vi "Compiled Get Node Settings.vi"(8 "error in":errorcluster, 10 "Cluster":refnum<k21>, 11 "Addon Ref":T21 format="%.0x") -> (0 "error out":errorcluster, 2 "J1939 Data Settings":T1 {"Monitor"."Data"."Outgoing"."Trigger.Refs"."Data Reference" format="%.0x"; "Monitor"."Data"."Outgoing"."Disable.Refs"."Data Reference" format="%.0x"; "Monitor"."Data"."Outgoing"."Data.Refs"."Data Reference" format="%.0x"; "Monitor"."Data"."Incoming"."Timing.Refs"."Data Reference" format="%.0x"; "Monitor"."Data"."Incoming"."Data.Refs"."Data Reference" format="%.0x"; "Monitor"."Network"."Name" format="%.0x"; "Sim"."DTCs"."DM1.Ref"."Data Reference" format="%.0x"; "Sim"."DTCs"."DM1.Enable.Ref"."Data Reference" format="%.0x"; "Sim"."DTCs"."DM2.Ref"."Data Reference" format="%.0x"; "Sim"."DTCs"."DM2.Enable.Ref"."Data Reference" format="%.0x"; "Sim"."Network"."Name" format="%.0x"}, 3 "Addon Ref out":T21=18446744073709551615 format="%.0x")   [LabVIEW 2023, in "J1939 Addon System Explorer.lvlib"]
uses:
  J1939 Addon System Explorer.lvlib
  <vilib>/NI VeriStand/Custom Device API/Custom Device Item Ref.ctl
  Addon Shared/Types/Compiled.Node Settings.ctl
  Addon Shared/Types/Compiled Monitor Tool Settings.ctl
  Addon Shared/Types/Monitor Settings.ctl
  Addon Shared/Types/Device Settings.ctl
  Addon Shared/Types/Incoming Settings.ctl
  Addon Shared/Types/Incoming Frame Settings.ctl
  <vilib>/NI VeriStand/Custom Device API/Block Data Reference.ctl
  <vilib>/NI VeriStand/Custom Device API/Data Reference.ctl
  Addon Shared/Types/Outgoing Settings.ctl
  Addon Shared/Types/Outgoing Frame Settings.ctl
  Addon Shared/Types/Outgoing Event Trigger Types.ctl
  SubModules/Frame-Protection-Support/Source/Shared/Types/Exported Frame Settings.ctl
  SubModules/Frame-Protection-Support/Source/Shared/Types/Exported Frame Type.ctl
  SubModules/Frame-Protection-Support/Source/Shared/Types/Exported Protection Settings.ctl
  SubModules/Frame-Protection-Support/Source/Shared/Types/Protection Type.ctl
  SubModules/Frame-Protection-Support/Source/Shared/Types/XNET Signal Configuration.ctl
  SubModules/Frame-Protection-Support/Source/Shared/Types/Exported Counter Settings.ctl
  SubModules/Frame-Protection-Support/Source/Shared/Types/Exported Event Trigger Type.ctl
  Addon Shared/Types/Complied Simulated Device Settings.ctl
  Addon Shared/Types/Compiled Simulated Settings.ctl
  Addon Shared/J1939 Addon Shared.lvlib
  <vilib>/NI VeriStand/Custom Device API/Custom Device API.lvlib
  <vilib>/NI/NIVS Inline Async API/_Data Access System Explorer/Data Access System Explorer.lvlib
  SubModules/Frame-Protection-Support/Source/Shared/Protection and Counter Support Shared.lvlib
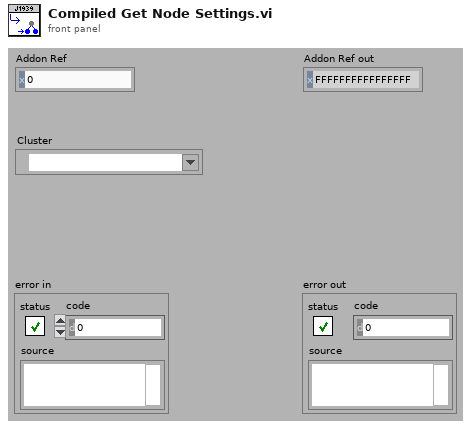
[diagram p1: front panel]
types:
  T1 = typedef "J1939 Addon Shared.lvlib/Compiled.Node Settings.ctl" = cluster{"Monitor":T2, "Sim":T19[]}
  T2 = typedef "J1939 Addon Shared.lvlib/Compiled Monitor Tool Settings.ctl" = cluster{"Network":T3, "Data":T4}
  T3 = typedef "J1939 Addon Shared.lvlib/Monitor Settings.ctl" = cluster{"Address":u8, "Name":u64, "Include DA":bool, "Force SA":bool}
  T4 = typedef "J1939 Addon Shared.lvlib/Device Settings.ctl" = cluster{"Incoming":T5, "Outgoing":T9}
  T5 = typedef "J1939 Addon Shared.lvlib/Incoming Settings.ctl" = cluster{"Signals":string[], "Frames":T6[], "Data.Refs":T7[], "Data.Values":dbl[], "Timing.Use":bool, "Timing.Refs":T7[], "Timing.Values":dbl[], "Timing.Index":i32[]}
  T6 = typedef "J1939 Addon Shared.lvlib/Incoming Frame Settings.ctl" = cluster{"Signals":string[], "PGN":u32}
  T7 = typedef "Custom Device API.lvlib/Block Data Reference.ctl" = cluster{"Data Reference":T8, "Offset":u64, "Length":u64}
  T8 = typedef "Custom Device API.lvlib/Data Reference.ctl" = i32
  T9 = typedef "J1939 Addon Shared.lvlib/Outgoing Settings.ctl" = cluster{"Frames":T10[], "Data.Refs":T7[], "Data.Values":dbl[], "Disable.Refs":T7[], "Disable.Values":dbl[], "Trigger.Refs":T7[], "Trigger.Values":dbl[], "Frames.CountersAndProtections":T12[]}
  T10 = typedef "J1939 Addon Shared.lvlib/Outgoing Frame Settings.ctl" = cluster{"Signals":string[], "Channel Array Position":cluster{"Offset":u32, "Length":u32}, "PGN":u32, "Cyclic?":bool, "Disable?":bool, "Disable.Index":i32, "Trigger":T11, "Trigger.Index":i32}
  T11 = typedef "J1939 Addon Shared.lvlib/Outgoing Event Trigger Types.ctl" = enum16{"Channel value change", "Trigger channel (not zero)", "Channel value change or trigger channel (not zero)", "Trigger channel (any value change)", "Channel value change or trigger channel (any value change)"}
  T12 = typedef "Protection and Counter Support Shared.lvlib/Exported Frame Settings.ctl" = cluster{"Type":T13, "Frame ID":u32, "Payload Length":u32, "Signal XNET Paths":string[], "Frame.PrevData":dbl[], "VS Offset":i32, "VS Length":i32, "Generation Period":u32, "Has Protection?":bool, "Protection Configurations":T14[], "Has Counter":bool, "Counter Configurations":T17[], "Has Disable?":bool, "Disable VS Index":i32, "Transmit Trigger":T18, "Trigger VS Index":i32}
  T13 = typedef "Protection and Counter Support Shared.lvlib/Exported Frame Type.ctl" = enum16{"Periodic", "Event", "Periodic/Event"}
  T14 = typedef "Protection and Counter Support Shared.lvlib/Exported Protection Settings.ctl" = cluster{"Protection Frame Index":i32, "Protection Type":T15, "Data Indeces":i32[], "Initialized Data Array":dbl[], "Protection Signal XNET Paths":string[], "CRC Channels":T16[], "Protection VS Update Index":i32, "Override Index":i32, "Override Value Index":i32}
  T15 = typedef "Protection and Counter Support Shared.lvlib/Protection Type.ctl" = enum16{"Arb ID + Bytes Checksum with Inversion", "Arb ID + Bytes CRC with Inversion", "Reversed Raw Signal Checksum with Inversion", "Concatenated Two's Compliment"}
  T16 = typedef "Protection and Counter Support Shared.lvlib/XNET Signal Configuration.ctl" = cluster{"Start Bit":i32, "Name":string, "Number of bits":i32, "Scale":dbl, "Offset":dbl, "Data Type":u32, "Counter":bool}
  T17 = typedef "Protection and Counter Support Shared.lvlib/Exported Counter Settings.ctl" = cluster{"Frame Index":i32, "Max Count":dbl, "VS Index":i32, "Bit Length":i64, "Override Index":i32, "Override Value Index":i32}
  T18 = typedef "Protection and Counter Support Shared.lvlib/Exported Event Trigger Type.ctl" = enum16{"Channel value change", "Trigger channel (not zero)", "Channel value change or trigger channel (not zero)", "Trigger channel (any value change)", "Channel value change or trigger channel (any value change)"}
  T19 = typedef "J1939 Addon Shared.lvlib/Complied Simulated Device Settings.ctl" = cluster{"Network":T3, "Data":T4, "DTCs":T20}
  T20 = typedef "J1939 Addon Shared.lvlib/Compiled Simulated Settings.ctl" = cluster{"DM1.Ref":T7[], "DM1.Value":dbl[], "DM1.Enable.Ref":T7[], "DM1.Enable.Value":dbl[], "DM2.Ref":T7[], "DM2.Value":dbl[], "DM2.Enable.Ref":T7[], "DM2.Enable.Value":dbl[]}
  T21 = typedef "Custom Device API.lvlib/Custom Device Item Ref.ctl" = u64
  T22 = cluster{"Name":string, "Type":enum16{"Output/Write", "Input/Read", "Input/ReadWrite"}, "VS Refs":T21[]}[]
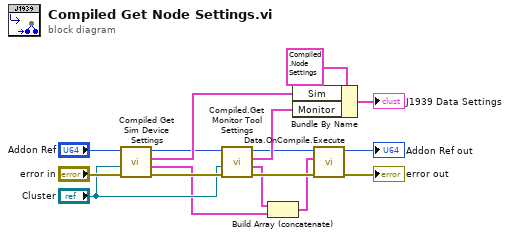
[diagram p0: block diagram]
diagram:
  n1 = call "Compiled Get Sim Device Settings.vi"("error in (no error)"="error in", "Cluster"="Cluster", "Addon Ref"="Addon Ref") -> ("error out"=w11:errorcluster, "Async Refs"=w3:T22, "Settings"=w13:T19[], "Addon Ref out"=w8:T21)  [unwired: 5 in]
  n2 = call "Compiled.Get Monitor Tool Settings.vi"("error in (no error)"=w11, "Cluster"="Cluster", "Addon Ref"=w8) -> ("error out"=w7:errorcluster, "VS Ref Groups"=w2:T22, "MonitorToolSettings"=w10:T2, "Addon Ref out"=w5:T21)  [unwired: 5 in]
  n3 = Build Array (concatenate)(w2, w3) -> (w1:T22)
  n4 = Bundle By Name(cluster=T1 {"Monitor"={"Network"={"Address"=0, "Name"=0, "Include DA"=FALSE, "Force SA"=FALSE}, "Data"={"Incoming"={"Signals"=[], "Frames"=[], "Data.Refs"=[], "Data.Values"=[], "Timing.Use"=FALSE, "Timing.Refs"=[], "Timing.Values"=[], "Timing.Index"=[]}, "Outgoing"={"Frames"=[], "Data.Refs"=[], "Data.Values"=[], "Disable.Refs"=[], "Disable.Values"=[], "Trigger.Refs"=[], "Trigger.Values"=[], "Frames.CountersAndProtections"=[]}}}, "Sim"=[]}, "Sim"=w13, "Monitor"=w10) -> (→"J1939 Data Settings":T1)
  n5 = call <vilib>:"Data.OnCompile.Execute.vi"("error in"=w7, "VS Ref Groups"=w1, "Custom Device Ref"=w5) -> ("error out"=→"error out":errorcluster, "Custom Device Ref"=→"Addon Ref out":T21)  [unwired: 7 in]
